vi "ClusterEscala.vi"() -> ()   [LabVIEW 2016]
panel:
  out "Cluster 3":T1 {"presion" scale=0.0..100.0; "flujo" scale=0.0..100.0; "temperatura" scale=0.0..100.0}
  out "Cluster 2":T2
  in  "Cluster":T3
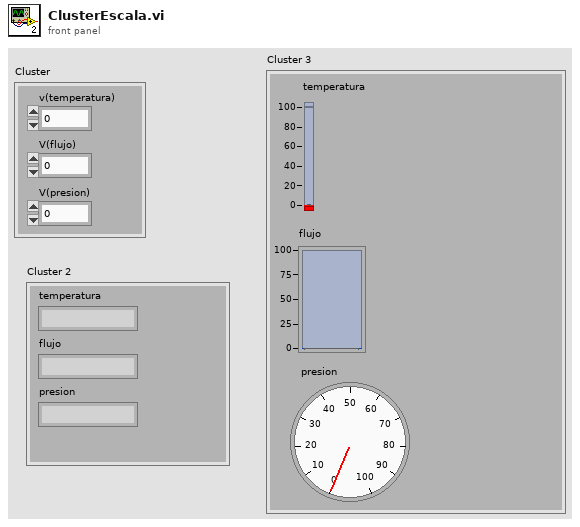
[diagram p1: front panel]
types:
  T1 = cluster{"temperatura":dbl, "flujo":dbl, "presion":dbl}
  T2 = cluster{"temperatura":string, "flujo":string, "presion":string}
  T3 = cluster{"V(presion)":dbl, "V(flujo)":dbl, "v(temperatura)":dbl}
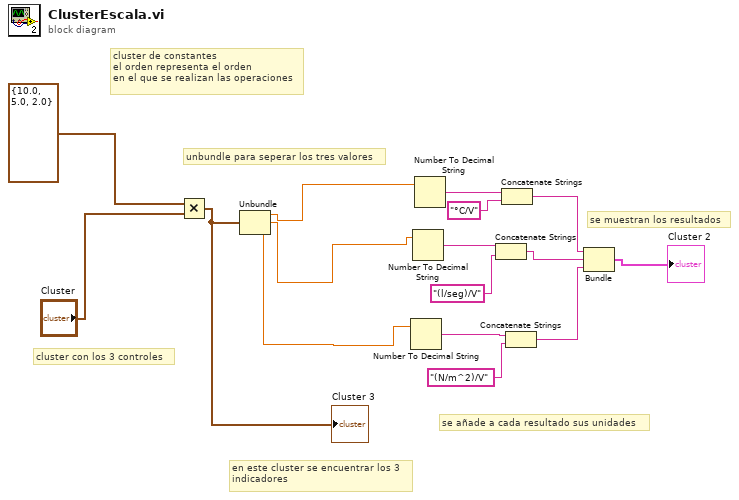
[diagram p0: block diagram]
diagram:
  # "en este cluster se encuentrar los 3 \nindicadores"
  # "se muestran los resultados"
  # "se añade a cada resultado sus unidades"
  # "unbundle para seperar los tres valores"
  # "cluster con los 3 controles"
  # "cluster de constantes \nel orden representa el orden \nen el que se realizan las operaciones"
  n1 = Multiply(x=cluster{dbl, dbl, dbl} {10.0, 5.0, 2.0}, y="Cluster") -> (x*y=w2:cluster{dbl, dbl, dbl})
  "Cluster 3" <- w2
  n2 = Unbundle(w2) -> (w15:dbl, w14:dbl, w13:dbl)
  n3 = Number To Decimal String(number=w13) -> (decimal integer string=w8:string)  [unwired: 1 in]
  n4 = Number To Decimal String(number=w14) -> (decimal integer string=w10:string)  [unwired: 1 in]
  n5 = Number To Decimal String(number=w15) -> (decimal integer string=w12:string)  [unwired: 1 in]
  n6 = Concatenate Strings(w10, "(l/seg)/V") -> (w5:string)
  n7 = Concatenate Strings(w12, "°C/V") -> (w6:string)
  n8 = Concatenate Strings(w8, "(N/m^2)/V") -> (w4:string)
  n9 = Bundle(w6, w5, w4) -> (→"Cluster 2":cluster{string, string, string})  [unwired: 1 in]
